vi "TrajectoryControllerAhead.vi"(0 "X":dbl, 5 "Y":dbl, 7 "Ahead":dbl format="%#_13g", 9 "Z":dbl, 11 "Trajectory":dbl[][](array[numeric])) -> (1 "error":cdb, 3 "XHD":dbl[](array[numeric]), 4 "Xclosest":dbl, 6 "Yclosest":dbl, 10 "Zclosest":dbl, 12 "ZHD":dbl[](array[numeric]), 14 "YHD":dbl[](array[numeric]), 15 "OptimumVelocity":dbl[](array[numeric]))   [LabVIEW 2020]
uses:
  <vilib>/imath/engines/lvmath2/RunTimeEngine/BuiltInFunctions/size/NIMS_[I32,I32]=size(GM).vi
  <instcachedir>/0/NIMS_[I32,I32]=size(GM)_B0A6EC1255BB4C8AB801FE6F734128D9.lvgen/NIMS_[I32,I32]=size(GM)_B0A6EC1255BB4C8AB801FE6F734128D9_000.vi
  <vilib>/imath/engines/lvmath2/RunTimeEngine/BuiltInFunctions/linramp/NIMS_linramp.vi
  <vilib>/imath/engines/lvmath2/RunTimeEngine/IndexRead/NIMS M($,S).vi
  <instcachedir>/0/NIMS M($,S)_3E5749BBB62E49528D4765A77F1F6D98.lvgen/NIMS M($,S)_3E5749BBB62E49528D4765A77F1F6D98_000.vi
  <vilib>/imath/engines/lvmath2/RunTimeEngine/BuiltInFunctions/interpolate1d/NIMS_interpolate1d(RV,RV,RV,Str).vi
  <vilib>/imath/engines/lvmath2/RunTimeEngine/ErrorHandling/NIMS_Create Error From Enums.vi
  <vilib>/imath/engines/lvmath2/RunTimeEngine/IndexRead/NIMS V(S).vi
  <instcachedir>/0/NIMS V(S)_0488751826AF41519A22953C041130DC.lvgen/NIMS V(S)_0488751826AF41519A22953C041130DC_000.vi
  <vilib>/imath/engines/lvmath2/RunTimeEngine/ArithmeticOperatorToken/NIMS_ArithmeticOperator_plus.vi
  <instcachedir>/0/NIMS_ArithmeticOperator_plus_54468E2FAC2848C4BF0D457641184E60.lvgen/NIMS_ArithmeticOperator_plus_54468E2FAC2848C4BF0D457641184E60_004.vi
  <vilib>/imath/engines/lvmath2/RunTimeEngine/BuiltInFunctions/min/1 input/NIMS_min(CV).vi
  <instcachedir>/0/NIMS_min(CV)_4AB3BA2E962D4964BA6C7B129334C4B7.lvgen/NIMS_min(CV)_4AB3BA2E962D4964BA6C7B129334C4B7_000.vi
  <vilib>/imath/engines/lvmath2/RunTimeEngine/BuiltInFunctions/length/NIMS_length(GV).vi
  <instcachedir>/0/NIMS_length(GV)_08A3D13377FD4E4B96F5795FBF3698FA.lvgen/NIMS_length(GV)_08A3D13377FD4E4B96F5795FBF3698FA_000.vi
  <vilib>/imath/engines/lvmath2/RunTimeEngine/VariableToken/NIMS_VariableToken_CondDefined.vi
  <instcachedir>/0/NIMS_VariableToken_CondDefined_537E119D71C74F9D9452D6FF923F1E1F.lvgen/NIMS_VariableToken_CondDefined_537E119D71C74F9D9452D6FF923F1E1F_003.vi
  <vilib>/imath/engines/lvmath2/RunTimeSupport/NIMS_Error if Not Equal.vi
  <instcachedir>/0/NIMS_Error if Not Equal_BE0C21F4A4FB4AC7AFE883167692CC6A.lvgen/NIMS_Error if Not Equal_BE0C21F4A4FB4AC7AFE883167692CC6A_000.vi
  <vilib>/imathl/engines/lvmath/Functions/Error Handling/Create Error.vi
  <vilib>/imath/engines/lvmath2/RunTimeEngine/BuiltInFunctions/norm/NIMS_norm(GV,DBL).vi
  <instcachedir>/0/NIMS_norm(GV,DBL)_118B4CCB667A4D7498CD7C123070720C.lvgen/NIMS_norm(GV,DBL)_118B4CCB667A4D7498CD7C123070720C_000.vi
  <vilib>/imath/engines/lvmath/Functions/Error Handling/MergeErrorsWrapper.vi
  <vilib>/imath/engines/lvmath2/RunTimeEngine/NodeEndStatement/NIMS_NodeEndStatement_Output.vi
  <instcachedir>/0/NIMS_NodeEndStatement_Output_53EC0D466D134D7ABD903AC30B43404B.lvgen/NIMS_NodeEndStatement_Output_53EC0D466D134D7ABD903AC30B43404B_001.vi
  <instcachedir>/0/NIMS_NodeEndStatement_Output_53EC0D466D134D7ABD903AC30B43404B.lvgen/NIMS_NodeEndStatement_Output_53EC0D466D134D7ABD903AC30B43404B_005.vi
  <instcachedir>/0/NIMS_NodeEndStatement_Output_53EC0D466D134D7ABD903AC30B43404B.lvgen/NIMS_NodeEndStatement_Output_53EC0D466D134D7ABD903AC30B43404B_009.vi
  <vilib>/imath/engines/lvmath2/RunTimeEngine/ErrorHandling/NIMS_Finalize Error.vi
panel:
  out "IndexMin":dbl
  out "MinCol":dbl
  out "TargetPoint":dbl[](array[numeric])
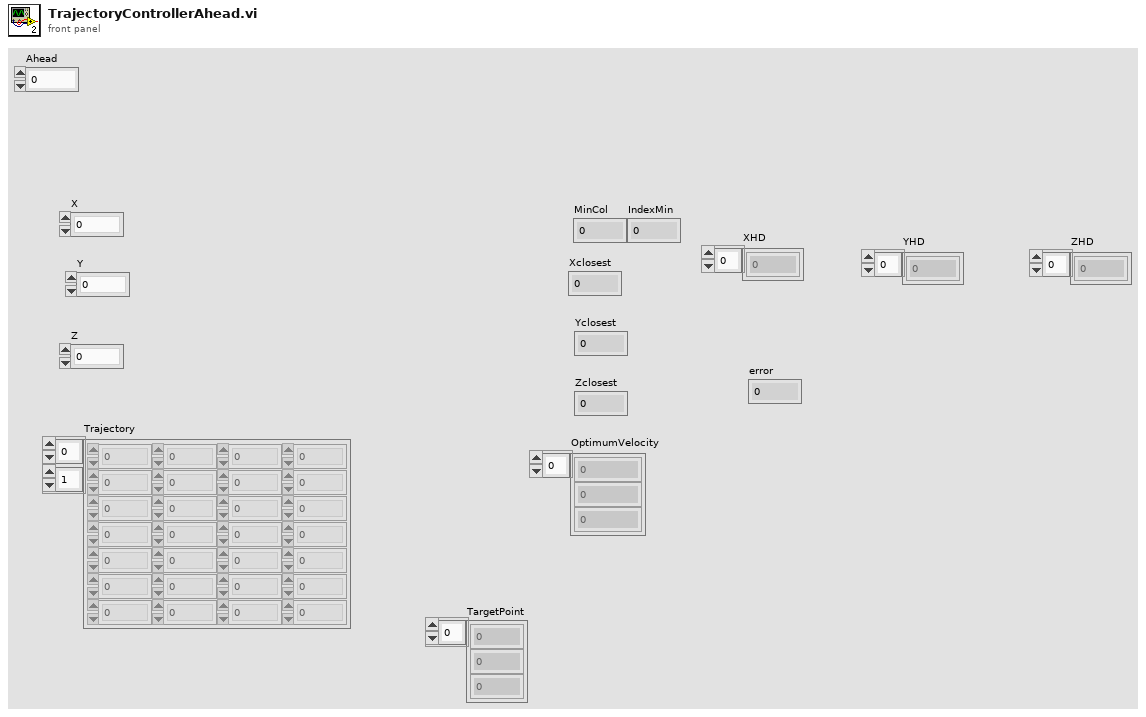
[diagram p1: front panel]
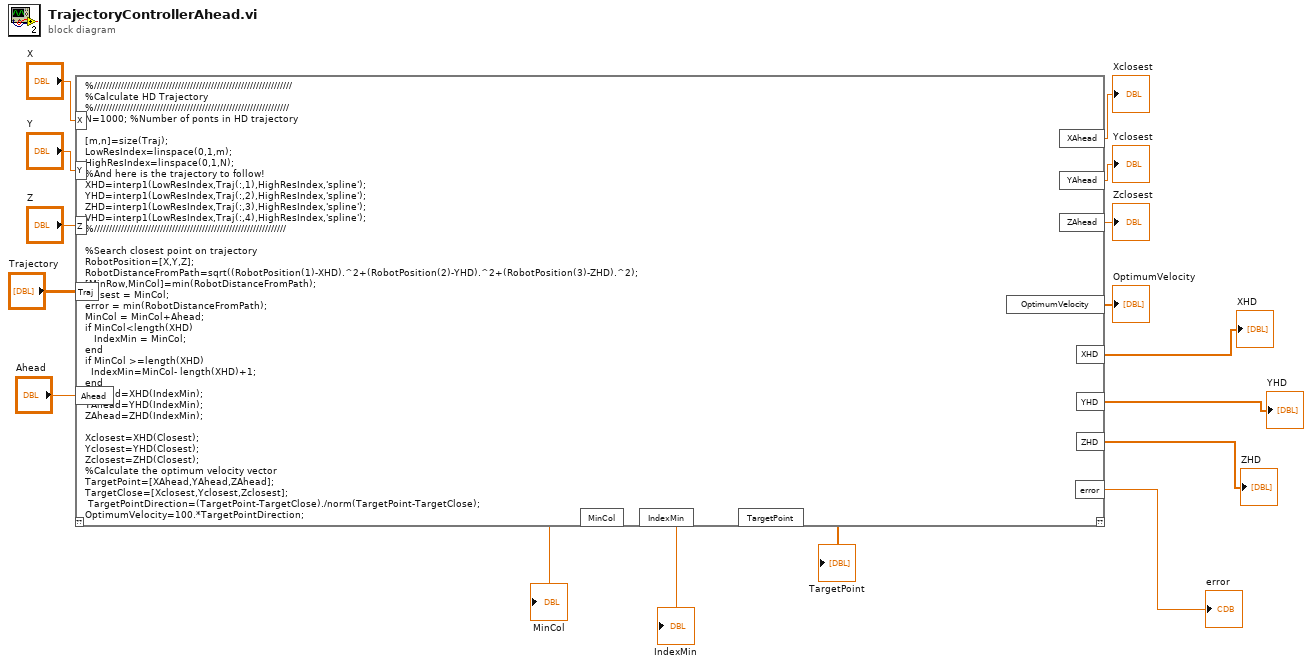
[diagram p0: block diagram]
diagram:
  n1 = mathscript code="%//////////////////////////////////////////////////////////////////\n%Calculate HD Trajectory\n%/////////////////////////////////////////////////////////////////\nN=1000; %Number of ponts in HD trajectory\n\n[m,n]=size(Traj);\nLowResIndex=linspace(0,1,m);\nHighResIndex=linspace(0,1,N);\n%And here is the trajectory to follow!\nXHD=interp1(LowResIndex,Traj(:,1),HighResIndex,'spline');\nYHD=interp1(LowResIndex,Traj(:,2),HighResIndex,'spline');\nZHD=interp1(LowResIndex,Traj(:,3),HighResIndex,'spline');\nVHD=interp1(LowResIndex,Traj(:,4),HighResIndex,'spline');\n%////////////////////////////////////////////////////////////////\n\n%Search closest point on trajectory\nRobotPosition=[X,Y,Z];\nRobotDistanceFromPath=sqrt((RobotPosition(1)-XHD).^2+(RobotPosition(2)-YHD).^2+(RobotPosition(3)-ZHD).^2);\n[MinRow,MinCol]=min(RobotDistanceFromPath);\nClosest = MinCol;\nerror = min(RobotDistanceFromPath);\nMinCol = MinCol+Ahead;\nif MinCol<length(XHD)\n   IndexMin = MinCol;\nend\nif MinCol >=length(XHD)\n  IndexMin=MinCol- length(XHD)+1;\nend\nXAhead=XHD(IndexMin);\nYAhead=YHD(IndexMin);\nZAhead=ZHD(IndexMin);\n\nXclosest=XHD(Closest);\nYclosest=YHD(Closest);\nZclosest=ZHD(Closest);\n%Calculate the optimum velocity vector\nTargetPoint=[XAhead,YAhead,ZAhead];\nTargetClose=[Xclosest,Yclosest,Zclosest];\n TargetPointDirection=(TargetPoint-TargetClose)./norm(TargetPoint-TargetClose);\nOptimumVelocity=100.*TargetPointDirection;"("X"="X", "Y"="Y", "Z"="Z", "Traj"="Trajectory", "Ahead"="Ahead") -> ("XAhead"=→"Xclosest":dbl, "YAhead"=→"Yclosest":dbl, "ZAhead"=→"Zclosest":dbl, "OptimumVelocity"=→"OptimumVelocity":dbl[], "XHD"=→"XHD":dbl[], "YHD"=→"YHD":dbl[], "ZHD"=→"ZHD":dbl[], "error"=→"error":cdb, "TargetPoint"=→"TargetPoint":dbl[], "MinCol"=→"MinCol":dbl, "IndexMin"=→"IndexMin":dbl)  [unwired: 1 in, 1 out]
